vi "ChargePump_DDR.vi"(8 "error in (no error)":errorcluster, 11 "Charge Pump Setting":string(combo)="Normal") -> (0 "error out":errorcluster)   [LabVIEW 2011]
doc: "This VI sets the charge pump to the desired state for the DDR PLL.\n\nInputs:\n1. Charge Pump Setting: Sets the charge pump to the desire state (Normal or Down)."
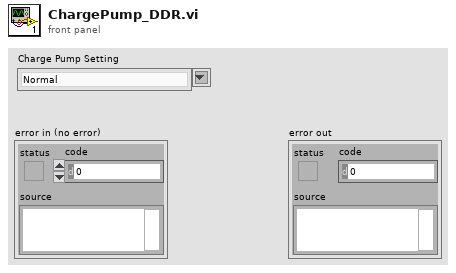
[diagram p1: front panel]
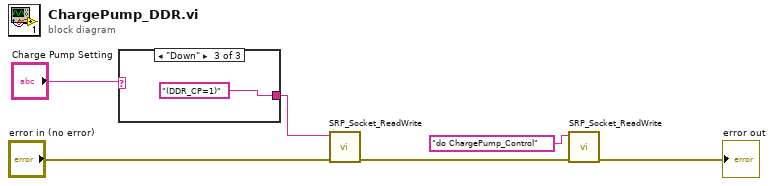
[diagram p0: block diagram]
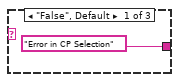
[diagram p2: hidden frame]
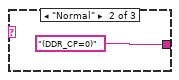
[diagram p3: hidden frame]
diagram:
  n1 = case shown="\"Down\"" "Charge Pump Setting" {
    tunnel: ["Error in CP Selection" "(DDR_CP=0)" "(DDR_CP=1)"] -> w3
    frame "False", Default {
    }
    frame "Normal" {
    }
    frame "Down" {
    }
  }
  n2 = call "SRP_Socket_ReadWrite.vi"("error in (no error)"="error in (no error)", "Data In"=w3) -> ("error out"=w4:errorcluster)  [unwired: 7 in, 1 out]
  n3 = call "SRP_Socket_ReadWrite.vi"("error in (no error)"=w4, "Data In"="do ChargePump_Control") -> ("error out"=→"error out":errorcluster)  [unwired: 7 in, 1 out]
